vi "NF WF1973_74 VI Tree.vi"   [LabVIEW 2010]
panel:
  # "Please display diagram\n to refer to VI Tree. \nShort-cut \"Ctrl+E\""
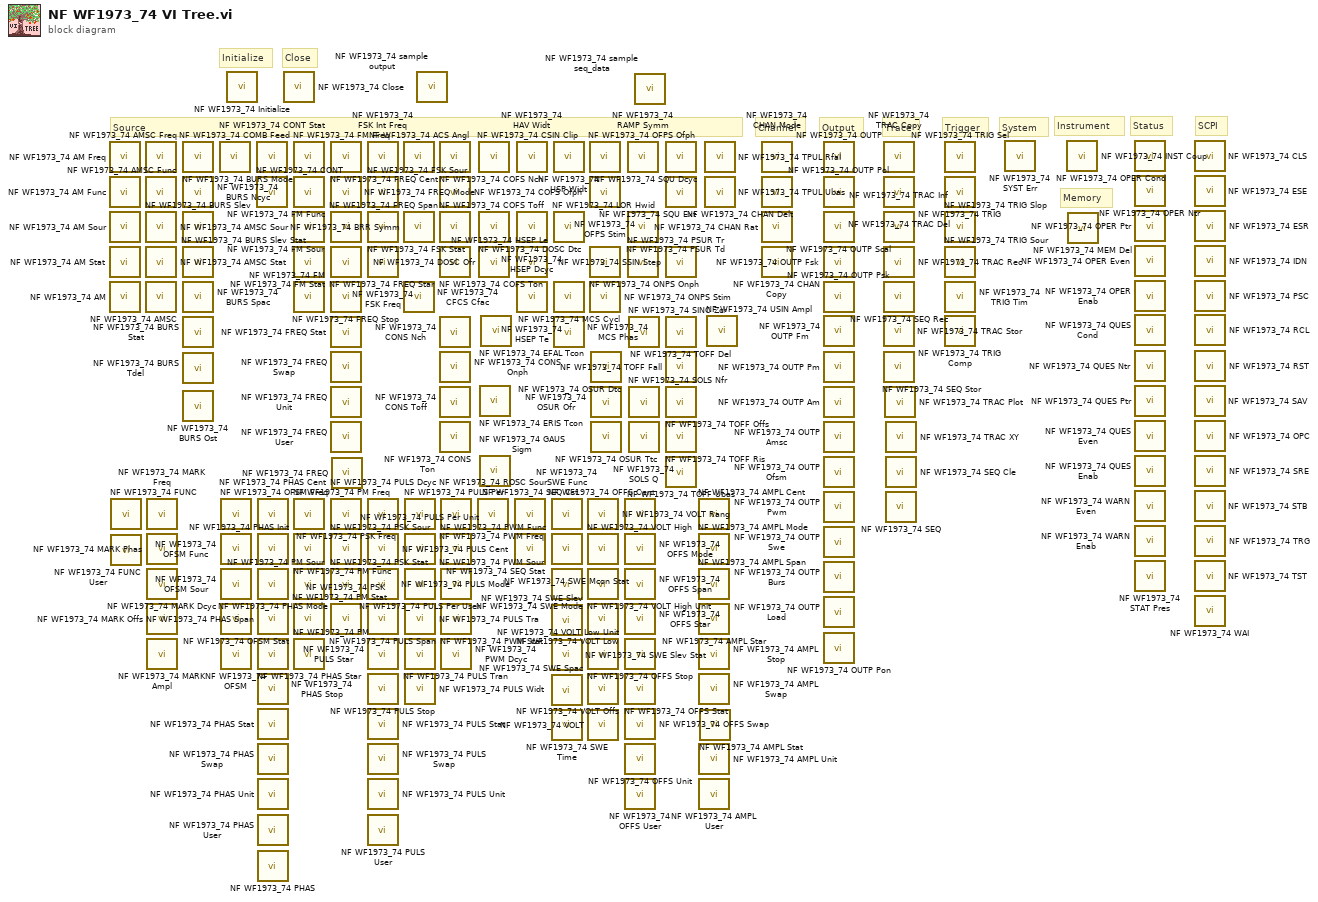
[diagram p0: block diagram]
diagram:
  # "SCPI"
  # "Status"
  # "Memory"
  # "Instrument"
  # "Trace"
  # "System"
  # "Trigger"
  # "Output"
  # "Channel"
  # "Close"
  # "Initialize"
  # "Source"
  n1 = call <instrlib>:"NF WF1973_74 AM Freq.vi"() -> ()  [unwired: 9 in, 3 out]
  n2 = call <instrlib>:"NF WF1973_74 AM Func.vi"() -> ()  [unwired: 9 in, 3 out]
  n3 = call <instrlib>:"NF WF1973_74 AM Sour.vi"() -> ()  [unwired: 9 in, 3 out]
  n4 = call <instrlib>:"NF WF1973_74 AM Stat.vi"() -> ()  [unwired: 9 in, 3 out]
  n5 = call <instrlib>:"NF WF1973_74 AM.vi"() -> ()  [unwired: 9 in, 3 out]
  n6 = call <instrlib>:"NF WF1973_74 FUNC.vi"() -> ()  [unwired: 9 in, 3 out]
  n7 = call <instrlib>:"NF WF1973_74 FUNC User.vi"() -> ()  [unwired: 9 in, 3 out]
  n8 = call <instrlib>:"NF WF1973_74 AMSC Freq.vi"() -> ()  [unwired: 9 in, 3 out]
  n9 = call <instrlib>:"NF WF1973_74 AMSC Func.vi"() -> ()  [unwired: 9 in, 3 out]
  n10 = call <instrlib>:"NF WF1973_74 AMSC Sour.vi"() -> ()  [unwired: 9 in, 3 out]
  n11 = call <instrlib>:"NF WF1973_74 AMSC Stat.vi"() -> ()  [unwired: 9 in, 3 out]
  n12 = call <instrlib>:"NF WF1973_74 AMSC.vi"() -> ()  [unwired: 9 in, 3 out]
  n13 = call <instrlib>:"NF WF1973_74 MARK Freq.vi"() -> ()  [unwired: 9 in, 3 out]
  n14 = call <instrlib>:"NF WF1973_74 MARK Phas.vi"() -> ()  [unwired: 9 in, 3 out]
  n15 = call <instrlib>:"NF WF1973_74 MARK Dcyc.vi"() -> ()  [unwired: 9 in, 3 out]
  n16 = call <instrlib>:"NF WF1973_74 MARK Offs.vi"() -> ()  [unwired: 9 in, 3 out]
  n17 = call <instrlib>:"NF WF1973_74 MARK Ampl.vi"() -> ()  [unwired: 9 in, 3 out]
  n18 = call <instrlib>:"NF WF1973_74 BURS Mode.vi"() -> ()  [unwired: 9 in, 3 out]
  n19 = call <instrlib>:"NF WF1973_74 BURS Ncyc.vi"() -> ()  [unwired: 9 in, 3 out]
  n20 = call <instrlib>:"NF WF1973_74 BURS Slev.vi"() -> ()  [unwired: 9 in, 3 out]
  n21 = call <instrlib>:"NF WF1973_74 BURS Slev Stat.vi"() -> ()  [unwired: 9 in, 3 out]
  n22 = call <instrlib>:"NF WF1973_74 BURS Spac.vi"() -> ()  [unwired: 9 in, 3 out]
  n23 = call <instrlib>:"NF WF1973_74 BURS Stat.vi"() -> ()  [unwired: 9 in, 3 out]
  n24 = call <instrlib>:"NF WF1973_74 BURS Tdel.vi"() -> ()  [unwired: 9 in, 3 out]
  n25 = call <instrlib>:"NF WF1973_74 BURS Ost.vi"() -> ()  [unwired: 9 in, 3 out]
  n26 = call <instrlib>:"NF WF1973_74 COMB Feed.vi"() -> ()  [unwired: 9 in, 3 out]
  n27 = call <instrlib>:"NF WF1973_74 OFSM Freq.vi"() -> ()  [unwired: 9 in, 3 out]
  n28 = call <instrlib>:"NF WF1973_74 OFSM Func.vi"() -> ()  [unwired: 9 in, 3 out]
  n29 = call <instrlib>:"NF WF1973_74 OFSM Sour.vi"() -> ()  [unwired: 9 in, 3 out]
  n30 = call <instrlib>:"NF WF1973_74 OFSM Stat.vi"() -> ()  [unwired: 9 in, 3 out]
  n31 = call <instrlib>:"NF WF1973_74 OFSM.vi"() -> ()  [unwired: 9 in, 3 out]
  n32 = call <instrlib>:"NF WF1973_74 Initialize.vi"() -> ()  [unwired: 4 in, 2 out]
  n33 = call <instrlib>:"NF WF1973_74 CONT Stat.vi"() -> ()  [unwired: 9 in, 3 out]
  n34 = call <instrlib>:"NF WF1973_74 CONT.vi"() -> ()  [unwired: 10 in, 2 out]
  n35 = call <instrlib>:"NF WF1973_74 PHAS Cent.vi"() -> ()  [unwired: 9 in, 3 out]
  n36 = call <instrlib>:"NF WF1973_74 PHAS Init.vi"() -> ()  [unwired: 10 in, 2 out]
  n37 = call <instrlib>:"NF WF1973_74 PHAS Mode.vi"() -> ()  [unwired: 9 in, 3 out]
  n38 = call <instrlib>:"NF WF1973_74 PHAS Span.vi"() -> ()  [unwired: 9 in, 3 out]
  n39 = call <instrlib>:"NF WF1973_74 PHAS Star.vi"() -> ()  [unwired: 9 in, 3 out]
  n40 = call <instrlib>:"NF WF1973_74 PHAS Stop.vi"() -> ()  [unwired: 9 in, 3 out]
  n41 = call <instrlib>:"NF WF1973_74 PHAS Stat.vi"() -> ()  [unwired: 10 in, 2 out]
  n42 = call <instrlib>:"NF WF1973_74 PHAS Swap.vi"() -> ()  [unwired: 10 in, 2 out]
  n43 = call <instrlib>:"NF WF1973_74 PHAS Unit.vi"() -> ()  [unwired: 9 in, 3 out]
  n44 = call <instrlib>:"NF WF1973_74 PHAS User.vi"() -> ()  [unwired: 13 in, 3 out]
  n45 = call <instrlib>:"NF WF1973_74 PHAS.vi"() -> ()  [unwired: 9 in, 3 out]
  n46 = call <instrlib>:"NF WF1973_74 Close.vi"() -> ()  [unwired: 2 in, 1 out]
  n47 = call <instrlib>:"NF WF1973_74 FM Freq.vi"() -> ()  [unwired: 9 in, 3 out]
  n48 = call <instrlib>:"NF WF1973_74 FM Func.vi"() -> ()  [unwired: 9 in, 3 out]
  n49 = call <instrlib>:"NF WF1973_74 FM Sour.vi"() -> ()  [unwired: 9 in, 3 out]
  n50 = call <instrlib>:"NF WF1973_74 FM Stat.vi"() -> ()  [unwired: 9 in, 3 out]
  n51 = call <instrlib>:"NF WF1973_74 FM.vi"() -> ()  [unwired: 9 in, 3 out]
  n52 = call <instrlib>:"NF WF1973_74 PM Freq.vi"() -> ()  [unwired: 9 in, 3 out]
  n53 = call <instrlib>:"NF WF1973_74 PM Func.vi"() -> ()  [unwired: 9 in, 3 out]
  n54 = call <instrlib>:"NF WF1973_74 PM Sour.vi"() -> ()  [unwired: 9 in, 3 out]
  n55 = call <instrlib>:"NF WF1973_74 PM Stat.vi"() -> ()  [unwired: 9 in, 3 out]
  n56 = call <instrlib>:"NF WF1973_74 PM.vi"() -> ()  [unwired: 9 in, 3 out]
  n57 = call <instrlib>:"NF WF1973_74 FREQ Cent.vi"() -> ()  [unwired: 9 in, 3 out]
  n58 = call <instrlib>:"NF WF1973_74 FREQ Mode.vi"() -> ()  [unwired: 9 in, 3 out]
  n59 = call <instrlib>:"NF WF1973_74 FREQ Span.vi"() -> ()  [unwired: 9 in, 3 out]
  n60 = call <instrlib>:"NF WF1973_74 FREQ Star.vi"() -> ()  [unwired: 9 in, 3 out]
  n61 = call <instrlib>:"NF WF1973_74 FREQ Stop.vi"() -> ()  [unwired: 9 in, 3 out]
  n62 = call <instrlib>:"NF WF1973_74 FREQ Stat.vi"() -> ()  [unwired: 11 in, 1 out]
  n63 = call <instrlib>:"NF WF1973_74 FREQ Swap.vi"() -> ()  [unwired: 10 in, 2 out]
  n64 = call <instrlib>:"NF WF1973_74 FREQ Unit.vi"() -> ()  [unwired: 9 in, 3 out]
  n65 = call <instrlib>:"NF WF1973_74 FREQ User.vi"() -> ()  [unwired: 13 in, 3 out]
  n66 = call <instrlib>:"NF WF1973_74 PSK Freq.vi"() -> ()  [unwired: 9 in, 3 out]
  n67 = call <instrlib>:"NF WF1973_74 PSK Sour.vi"() -> ()  [unwired: 9 in, 3 out]
  n68 = call <instrlib>:"NF WF1973_74 PSK Stat.vi"() -> ()  [unwired: 9 in, 3 out]
  n69 = call <instrlib>:"NF WF1973_74 PSK.vi"() -> ()  [unwired: 9 in, 3 out]
  n70 = call <instrlib>:"NF WF1973_74 FREQ.vi"() -> ()  [unwired: 9 in, 3 out]
  n71 = call <instrlib>:"NF WF1973_74 FSK Int Freq.vi"() -> ()  [unwired: 9 in, 3 out]
  n72 = call <instrlib>:"NF WF1973_74 FSK Sour.vi"() -> ()  [unwired: 9 in, 3 out]
  n73 = call <instrlib>:"NF WF1973_74 FSK Stat.vi"() -> ()  [unwired: 9 in, 3 out]
  n74 = call <instrlib>:"NF WF1973_74 FSK Freq.vi"() -> ()  [unwired: 9 in, 3 out]
  n75 = call <instrlib>:"NF WF1973_74 PULS Dcyc.vi"() -> ()  [unwired: 9 in, 3 out]
  n76 = call <instrlib>:"NF WF1973_74 PULS Cent.vi"() -> ()  [unwired: 9 in, 3 out]
  n77 = call <instrlib>:"NF WF1973_74 PULS Mode.vi"() -> ()  [unwired: 9 in, 3 out]
  n78 = call <instrlib>:"NF WF1973_74 PULS Span.vi"() -> ()  [unwired: 9 in, 3 out]
  n79 = call <instrlib>:"NF WF1973_74 PULS Star.vi"() -> ()  [unwired: 9 in, 3 out]
  n80 = call <instrlib>:"NF WF1973_74 PULS Stop.vi"() -> ()  [unwired: 9 in, 3 out]
  n81 = call <instrlib>:"NF WF1973_74 PULS Stat.vi"() -> ()  [unwired: 10 in, 2 out]
  n82 = call <instrlib>:"NF WF1973_74 PULS Swap.vi"() -> ()  [unwired: 10 in, 2 out]
  n83 = call <instrlib>:"NF WF1973_74 PULS Unit.vi"() -> ()  [unwired: 9 in, 3 out]
  n84 = call <instrlib>:"NF WF1973_74 PULS User.vi"() -> ()  [unwired: 13 in, 3 out]
  n85 = call <instrlib>:"NF WF1973_74 ACS Angl.vi"() -> ()  [unwired: 9 in, 3 out]
  n86 = call <instrlib>:"NF WF1973_74 BRR Symm.vi"() -> ()  [unwired: 9 in, 3 out]
  n87 = call <instrlib>:"NF WF1973_74 CFCS Cfac.vi"() -> ()  [unwired: 9 in, 3 out]
  n88 = call <instrlib>:"NF WF1973_74 PULS Per.vi"() -> ()  [unwired: 9 in, 3 out]
  n89 = call <instrlib>:"NF WF1973_74 PULS Per Unit.vi"() -> ()  [unwired: 9 in, 3 out]
  n90 = call <instrlib>:"NF WF1973_74 PULS Per User.vi"() -> ()  [unwired: 13 in, 3 out]
  n91 = call <instrlib>:"NF WF1973_74 PULS Tra.vi"() -> ()  [unwired: 9 in, 3 out]
  n92 = call <instrlib>:"NF WF1973_74 PULS Tran.vi"() -> ()  [unwired: 9 in, 3 out]
  n93 = call <instrlib>:"NF WF1973_74 PULS Widt.vi"() -> ()  [unwired: 9 in, 3 out]
  n94 = call <instrlib>:"NF WF1973_74 sample output.vi"() -> ()  [unwired: 14 in, 2 out]
  n95 = call <instrlib>:"NF WF1973_74 COFS Nch.vi"() -> ()  [unwired: 9 in, 3 out]
  n96 = call <instrlib>:"NF WF1973_74 COFS Ofph.vi"() -> ()  [unwired: 9 in, 3 out]
  n97 = call <instrlib>:"NF WF1973_74 COFS Toff.vi"() -> ()  [unwired: 9 in, 3 out]
  n98 = call <instrlib>:"NF WF1973_74 COFS Ton.vi"() -> ()  [unwired: 9 in, 3 out]
  n99 = call <instrlib>:"NF WF1973_74 CONS Nch.vi"() -> ()  [unwired: 9 in, 3 out]
  n100 = call <instrlib>:"NF WF1973_74 CONS Onph.vi"() -> ()  [unwired: 9 in, 3 out]
  n101 = call <instrlib>:"NF WF1973_74 CONS Toff.vi"() -> ()  [unwired: 9 in, 3 out]
  n102 = call <instrlib>:"NF WF1973_74 CONS Ton.vi"() -> ()  [unwired: 9 in, 3 out]
  n103 = call <instrlib>:"NF WF1973_74 PWM Freq.vi"() -> ()  [unwired: 9 in, 3 out]
  n104 = call <instrlib>:"NF WF1973_74 PWM Func.vi"() -> ()  [unwired: 9 in, 3 out]
  n105 = call <instrlib>:"NF WF1973_74 PWM Sour.vi"() -> ()  [unwired: 9 in, 3 out]
  n106 = call <instrlib>:"NF WF1973_74 PWM Stat.vi"() -> ()  [unwired: 9 in, 3 out]
  n107 = call <instrlib>:"NF WF1973_74 PWM Dcyc.vi"() -> ()  [unwired: 9 in, 3 out]
  n108 = call <instrlib>:"NF WF1973_74 ROSC Sour.vi"() -> ()  [unwired: 9 in, 3 out]
  n109 = call <instrlib>:"NF WF1973_74 CSIN Clip.vi"() -> ()  [unwired: 9 in, 3 out]
  n110 = call <instrlib>:"NF WF1973_74 DOSC Dtc.vi"() -> ()  [unwired: 9 in, 3 out]
  n111 = call <instrlib>:"NF WF1973_74 DOSC Ofr.vi"() -> ()  [unwired: 9 in, 3 out]
  n112 = call <instrlib>:"NF WF1973_74 ERIS Tcon.vi"() -> ()  [unwired: 9 in, 3 out]
  n113 = call <instrlib>:"NF WF1973_74 GAUS Sigm.vi"() -> ()  [unwired: 9 in, 3 out]
  n114 = call <instrlib>:"NF WF1973_74 EFAL Tcon.vi"() -> ()  [unwired: 9 in, 3 out]
  n115 = call <instrlib>:"NF WF1973_74 SEQ Cst.vi"() -> ()  [unwired: 9 in, 3 out]
  n116 = call <instrlib>:"NF WF1973_74 SEQ Stat.vi"() -> ()  [unwired: 9 in, 3 out]
  n117 = call <instrlib>:"NF WF1973_74 HAV Widt.vi"() -> ()  [unwired: 9 in, 3 out]
  n118 = call <instrlib>:"NF WF1973_74 HSEP Dcyc.vi"() -> ()  [unwired: 9 in, 3 out]
  n119 = call <instrlib>:"NF WF1973_74 HSEP Le.vi"() -> ()  [unwired: 9 in, 3 out]
  n120 = call <instrlib>:"NF WF1973_74 HSEP Te.vi"() -> ()  [unwired: 9 in, 3 out]
  n121 = call <instrlib>:"NF WF1973_74 SWE Func.vi"() -> ()  [unwired: 9 in, 3 out]
  n122 = call <instrlib>:"NF WF1973_74 SWE Mcon Stat.vi"() -> ()  [unwired: 9 in, 3 out]
  n123 = call <instrlib>:"NF WF1973_74 SWE Mode.vi"() -> ()  [unwired: 9 in, 3 out]
  n124 = call <instrlib>:"NF WF1973_74 SWE Slev.vi"() -> ()  [unwired: 9 in, 3 out]
  n125 = call <instrlib>:"NF WF1973_74 SWE Slev Stat.vi"() -> ()  [unwired: 9 in, 3 out]
  n126 = call <instrlib>:"NF WF1973_74 SWE Spac.vi"() -> ()  [unwired: 9 in, 3 out]
  n127 = call <instrlib>:"NF WF1973_74 SWE Time.vi"() -> ()  [unwired: 9 in, 3 out]
  n128 = call <instrlib>:"NF WF1973_74 HSP Widt.vi"() -> ()  [unwired: 9 in, 3 out]
  n129 = call <instrlib>:"NF WF1973_74 LOR Hwid.vi"() -> ()  [unwired: 9 in, 3 out]
  n130 = call <instrlib>:"NF WF1973_74 MCS Cycl.vi"() -> ()  [unwired: 9 in, 3 out]
  n131 = call <instrlib>:"NF WF1973_74 MCS Phas.vi"() -> ()  [unwired: 9 in, 3 out]
  n132 = call <instrlib>:"NF WF1973_74 VOLT Rang.vi"() -> ()  [unwired: 9 in, 3 out]
  n133 = call <instrlib>:"NF WF1973_74 VOLT High.vi"() -> ()  [unwired: 9 in, 3 out]
  n134 = call <instrlib>:"NF WF1973_74 VOLT High Unit.vi"() -> ()  [unwired: 9 in, 3 out]
  n135 = call <instrlib>:"NF WF1973_74 VOLT Low.vi"() -> ()  [unwired: 9 in, 3 out]
  n136 = call <instrlib>:"NF WF1973_74 VOLT Low Unit.vi"() -> ()  [unwired: 9 in, 3 out]
  n137 = call <instrlib>:"NF WF1973_74 VOLT Offs.vi"() -> ()  [unwired: 9 in, 3 out]
  n138 = call <instrlib>:"NF WF1973_74 VOLT.vi"() -> ()  [unwired: 9 in, 3 out]
  n139 = call <instrlib>:"NF WF1973_74 OFPS Ofph.vi"() -> ()  [unwired: 9 in, 3 out]
  n140 = call <instrlib>:"NF WF1973_74 OFPS Stim.vi"() -> ()  [unwired: 9 in, 3 out]
  n141 = call <instrlib>:"NF WF1973_74 ONPS Onph.vi"() -> ()  [unwired: 9 in, 3 out]
  n142 = call <instrlib>:"NF WF1973_74 ONPS Stim.vi"() -> ()  [unwired: 9 in, 3 out]
  n143 = call <instrlib>:"NF WF1973_74 OSUR Dtc.vi"() -> ()  [unwired: 9 in, 3 out]
  n144 = call <instrlib>:"NF WF1973_74 OSUR Ofr.vi"() -> ()  [unwired: 9 in, 3 out]
  n145 = call <instrlib>:"NF WF1973_74 OSUR Ttc.vi"() -> ()  [unwired: 9 in, 3 out]
  n146 = call <instrlib>:"NF WF1973_74 OFFS Cent.vi"() -> ()  [unwired: 9 in, 3 out]
  n147 = call <instrlib>:"NF WF1973_74 OFFS Mode.vi"() -> ()  [unwired: 9 in, 3 out]
  n148 = call <instrlib>:"NF WF1973_74 OFFS Span.vi"() -> ()  [unwired: 9 in, 3 out]
  n149 = call <instrlib>:"NF WF1973_74 OFFS Star.vi"() -> ()  [unwired: 9 in, 3 out]
  n150 = call <instrlib>:"NF WF1973_74 OFFS Stop.vi"() -> ()  [unwired: 9 in, 3 out]
  n151 = call <instrlib>:"NF WF1973_74 OFFS Stat.vi"() -> ()  [unwired: 10 in, 2 out]
  n152 = call <instrlib>:"NF WF1973_74 OFFS Swap.vi"() -> ()  [unwired: 10 in, 2 out]
  n153 = call <instrlib>:"NF WF1973_74 OFFS Unit.vi"() -> ()  [unwired: 9 in, 3 out]
  n154 = call <instrlib>:"NF WF1973_74 OFFS User.vi"() -> ()  [unwired: 13 in, 3 out]
  n155 = call <instrlib>:"NF WF1973_74 RAMP Symm.vi"() -> ()  [unwired: 9 in, 3 out]
  n156 = call <instrlib>:"NF WF1973_74 PSUR Td.vi"() -> ()  [unwired: 9 in, 3 out]
  n157 = call <instrlib>:"NF WF1973_74 PSUR Tr.vi"() -> ()  [unwired: 9 in, 3 out]
  n158 = call <instrlib>:"NF WF1973_74 SINC Zcr.vi"() -> ()  [unwired: 9 in, 3 out]
  n159 = call <instrlib>:"NF WF1973_74 SOLS Nfr.vi"() -> ()  [unwired: 9 in, 3 out]
  n160 = call <instrlib>:"NF WF1973_74 SOLS Q.vi"() -> ()  [unwired: 9 in, 3 out]
  n161 = call <instrlib>:"NF WF1973_74 sample seq_data.vi"() -> ()  [unwired: 1 in]
  n162 = call <instrlib>:"NF WF1973_74 SQU Dcyc.vi"() -> ()  [unwired: 9 in, 3 out]
  n163 = call <instrlib>:"NF WF1973_74 SQU Ext.vi"() -> ()  [unwired: 9 in, 3 out]
  n164 = call <instrlib>:"NF WF1973_74 SSIN Step.vi"() -> ()  [unwired: 9 in, 3 out]
  n165 = call <instrlib>:"NF WF1973_74 TOFF Del.vi"() -> ()  [unwired: 9 in, 3 out]
  n166 = call <instrlib>:"NF WF1973_74 TOFF Fall.vi"() -> ()  [unwired: 9 in, 3 out]
  n167 = call <instrlib>:"NF WF1973_74 TOFF Offs.vi"() -> ()  [unwired: 9 in, 3 out]
  n168 = call <instrlib>:"NF WF1973_74 TOFF Ris.vi"() -> ()  [unwired: 9 in, 3 out]
  n169 = call <instrlib>:"NF WF1973_74 TOFF Ubas.vi"() -> ()  [unwired: 9 in, 3 out]
  n170 = call <instrlib>:"NF WF1973_74 AMPL Cent.vi"() -> ()  [unwired: 9 in, 3 out]
  n171 = call <instrlib>:"NF WF1973_74 AMPL Mode.vi"() -> ()  [unwired: 9 in, 3 out]
  n172 = call <instrlib>:"NF WF1973_74 AMPL Span.vi"() -> ()  [unwired: 9 in, 3 out]
  n173 = call <instrlib>:"NF WF1973_74 AMPL Star.vi"() -> ()  [unwired: 9 in, 3 out]
  n174 = call <instrlib>:"NF WF1973_74 AMPL Stop.vi"() -> ()  [unwired: 9 in, 3 out]
  n175 = call <instrlib>:"NF WF1973_74 AMPL Swap.vi"() -> ()  [unwired: 10 in, 2 out]
  n176 = call <instrlib>:"NF WF1973_74 AMPL Unit.vi"() -> ()  [unwired: 9 in, 3 out]
  n177 = call <instrlib>:"NF WF1973_74 AMPL User.vi"() -> ()  [unwired: 13 in, 3 out]
  n178 = call <instrlib>:"NF WF1973_74 AMPL Stat.vi"() -> ()  [unwired: 10 in, 2 out]
  n179 = call <instrlib>:"NF WF1973_74 TPUL Rfal.vi"() -> ()  [unwired: 9 in, 3 out]
  n180 = call <instrlib>:"NF WF1973_74 TPUL Ubas.vi"() -> ()  [unwired: 9 in, 3 out]
  n181 = call <instrlib>:"NF WF1973_74 USIN Ampl.vi"() -> ()  [unwired: 9 in, 3 out]
  n182 = call <instrlib>:"NF WF1973_74 CHAN Mode.vi"() -> ()  [unwired: 9 in, 3 out]
  n183 = call <instrlib>:"NF WF1973_74 CHAN Delt.vi"() -> ()  [unwired: 13 in, 3 out]
  n184 = call <instrlib>:"NF WF1973_74 CHAN Rat.vi"() -> ()  [unwired: 13 in, 3 out]
  n185 = call <instrlib>:"NF WF1973_74 CHAN Copy.vi"() -> ()  [unwired: 10 in, 2 out]
  n186 = call <instrlib>:"NF WF1973_74 OUTP.vi"() -> ()  [unwired: 9 in, 3 out]
  n187 = call <instrlib>:"NF WF1973_74 OUTP Pol.vi"() -> ()  [unwired: 9 in, 3 out]
  n188 = call <instrlib>:"NF WF1973_74 OUTP Scal.vi"() -> ()  [unwired: 9 in, 3 out]
  n189 = call <instrlib>:"NF WF1973_74 OUTP Fsk.vi"() -> ()  [unwired: 9 in, 3 out]
  n190 = call <instrlib>:"NF WF1973_74 OUTP Psk.vi"() -> ()  [unwired: 9 in, 3 out]
  n191 = call <instrlib>:"NF WF1973_74 OUTP Fm.vi"() -> ()  [unwired: 9 in, 3 out]
  n192 = call <instrlib>:"NF WF1973_74 OUTP Pm.vi"() -> ()  [unwired: 9 in, 3 out]
  n193 = call <instrlib>:"NF WF1973_74 OUTP Am.vi"() -> ()  [unwired: 9 in, 3 out]
  n194 = call <instrlib>:"NF WF1973_74 OUTP Amsc.vi"() -> ()  [unwired: 9 in, 3 out]
  n195 = call <instrlib>:"NF WF1973_74 OUTP Ofsm.vi"() -> ()  [unwired: 9 in, 3 out]
  n196 = call <instrlib>:"NF WF1973_74 OUTP Pwm.vi"() -> ()  [unwired: 9 in, 3 out]
  n197 = call <instrlib>:"NF WF1973_74 OUTP Swe.vi"() -> ()  [unwired: 9 in, 3 out]
  n198 = call <instrlib>:"NF WF1973_74 OUTP Burs.vi"() -> ()  [unwired: 9 in, 3 out]
  n199 = call <instrlib>:"NF WF1973_74 OUTP Load.vi"() -> ()  [unwired: 9 in, 3 out]
  n200 = call <instrlib>:"NF WF1973_74 OUTP Pon.vi"() -> ()  [unwired: 9 in, 3 out]
  n201 = call <instrlib>:"NF WF1973_74 TRAC Copy.vi"() -> ()  [unwired: 10 in, 2 out]
  n202 = call <instrlib>:"NF WF1973_74 TRAC Del.vi"() -> ()  [unwired: 10 in, 2 out]
  n203 = call <instrlib>:"NF WF1973_74 TRAC Inf.vi"() -> ()  [unwired: 9 in, 3 out]
  n204 = call <instrlib>:"NF WF1973_74 TRAC Rec.vi"() -> ()  [unwired: 10 in, 2 out]
  n205 = call <instrlib>:"NF WF1973_74 SEQ Rec.vi"() -> ()  [unwired: 10 in, 2 out]
  n206 = call <instrlib>:"NF WF1973_74 TRAC Stor.vi"() -> ()  [unwired: 10 in, 2 out]
  n207 = call <instrlib>:"NF WF1973_74 SEQ Stor.vi"() -> ()  [unwired: 10 in, 2 out]
  n208 = call <instrlib>:"NF WF1973_74 TRAC Plot.vi"() -> ()  [unwired: 14 in, 2 out]
  n209 = call <instrlib>:"NF WF1973_74 TRAC XY.vi"() -> ()  [unwired: 14 in, 2 out]
  n210 = call <instrlib>:"NF WF1973_74 SEQ Cle.vi"() -> ()  [unwired: 10 in, 2 out]
  n211 = call <instrlib>:"NF WF1973_74 SEQ.vi"() -> ()  [unwired: 10 in, 2 out]
  n212 = call <instrlib>:"NF WF1973_74 TRIG Sel.vi"() -> ()  [unwired: 10 in, 2 out]
  n213 = call <instrlib>:"NF WF1973_74 TRIG.vi"() -> ()  [unwired: 10 in, 2 out]
  n214 = call <instrlib>:"NF WF1973_74 TRIG Slop.vi"() -> ()  [unwired: 9 in, 3 out]
  n215 = call <instrlib>:"NF WF1973_74 TRIG Sour.vi"() -> ()  [unwired: 9 in, 3 out]
  n216 = call <instrlib>:"NF WF1973_74 TRIG Tim.vi"() -> ()  [unwired: 9 in, 3 out]
  n217 = call <instrlib>:"NF WF1973_74 TRIG Comp.vi"() -> ()  [unwired: 10 in, 2 out]
  n218 = call <instrlib>:"NF WF1973_74 SYST Err.vi"() -> ()  [unwired: 3 in, 3 out]
  n219 = call <instrlib>:"NF WF1973_74 INST Coup.vi"() -> ()  [unwired: 9 in, 3 out]
  n220 = call <instrlib>:"NF WF1973_74 MEM Del.vi"() -> ()  [unwired: 10 in, 2 out]
  n221 = call <instrlib>:"NF WF1973_74 OPER Cond.vi"() -> ()  [unwired: 9 in, 3 out]
  n222 = call <instrlib>:"NF WF1973_74 OPER Ntr.vi"() -> ()  [unwired: 9 in, 3 out]
  n223 = call <instrlib>:"NF WF1973_74 OPER Ptr.vi"() -> ()  [unwired: 9 in, 3 out]
  n224 = call <instrlib>:"NF WF1973_74 OPER Even.vi"() -> ()  [unwired: 9 in, 3 out]
  n225 = call <instrlib>:"NF WF1973_74 OPER Enab.vi"() -> ()  [unwired: 9 in, 3 out]
  n226 = call <instrlib>:"NF WF1973_74 QUES Cond.vi"() -> ()  [unwired: 9 in, 3 out]
  n227 = call <instrlib>:"NF WF1973_74 QUES Ntr.vi"() -> ()  [unwired: 9 in, 3 out]
  n228 = call <instrlib>:"NF WF1973_74 QUES Ptr.vi"() -> ()  [unwired: 9 in, 3 out]
  n229 = call <instrlib>:"NF WF1973_74 QUES Even.vi"() -> ()  [unwired: 9 in, 3 out]
  n230 = call <instrlib>:"NF WF1973_74 QUES Enab.vi"() -> ()  [unwired: 9 in, 3 out]
  n231 = call <instrlib>:"NF WF1973_74 WARN Even.vi"() -> ()  [unwired: 9 in, 3 out]
  n232 = call <instrlib>:"NF WF1973_74 WARN Enab.vi"() -> ()  [unwired: 9 in, 3 out]
  n233 = call <instrlib>:"NF WF1973_74 STAT Pres.vi"() -> ()  [unwired: 10 in, 2 out]
  n234 = call <instrlib>:"NF WF1973_74 CLS.vi"() -> ()  [unwired: 10 in, 2 out]
  n235 = call <instrlib>:"NF WF1973_74 ESE.vi"() -> ()  [unwired: 9 in, 3 out]
  n236 = call <instrlib>:"NF WF1973_74 ESR.vi"() -> ()  [unwired: 9 in, 3 out]
  n237 = call <instrlib>:"NF WF1973_74 IDN.vi"() -> ()  [unwired: 9 in, 3 out]
  n238 = call <instrlib>:"NF WF1973_74 PSC.vi"() -> ()  [unwired: 9 in, 3 out]
  n239 = call <instrlib>:"NF WF1973_74 RCL.vi"() -> ()  [unwired: 10 in, 2 out]
  n240 = call <instrlib>:"NF WF1973_74 RST.vi"() -> ()  [unwired: 2 in, 2 out]
  n241 = call <instrlib>:"NF WF1973_74 SAV.vi"() -> ()  [unwired: 10 in, 2 out]
  n242 = call <instrlib>:"NF WF1973_74 OPC.vi"() -> ()  [unwired: 9 in, 3 out]
  n243 = call <instrlib>:"NF WF1973_74 SRE.vi"() -> ()  [unwired: 9 in, 3 out]
  n244 = call <instrlib>:"NF WF1973_74 STB.vi"() -> ()  [unwired: 9 in, 3 out]
  n245 = call <instrlib>:"NF WF1973_74 TRG.vi"() -> ()  [unwired: 10 in, 2 out]
  n246 = call <instrlib>:"NF WF1973_74 TST.vi"() -> ()  [unwired: 9 in, 3 out]
  n247 = call <instrlib>:"NF WF1973_74 WAI.vi"() -> ()  [unwired: 10 in, 2 out]
